vi "Test Multiply With Self.vi"(11 "Numeric":dbl) -> (3 "Gauge":dbl(knob) scale=0.0..10.0)   [LabVIEW 2024]
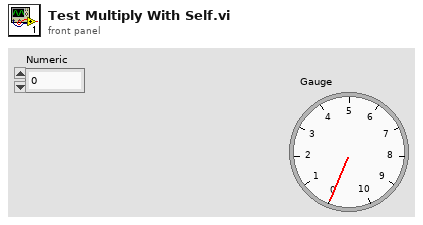
[diagram p1: front panel]
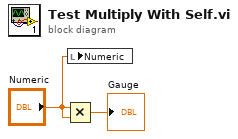
[diagram p0: block diagram]
diagram:
  n1 = Multiply(x="Numeric", y="Numeric") -> (x*y=→"Gauge":dbl)
  n2 = local write "Numeric"("Numeric") -> ()
